vi "Stop Motion.vi"(4 "error in (no error)":errorcluster, 5 "Stop all axes (F)":bool, 6 "Axis (1)":i32=1 min=1 max=3, 7 "VISA resource name":refnum<visa-resource-name>) -> (0 "error out":errorcluster, 3 "VISA resource name out":refnum<visa-resource-name>)   [LabVIEW 2012, in "Newport ESP301.lvlib"]
doc: "This command stops a motion in progress using deceleration rate programmed with AG (set deceleration) command on the specified axes (or all axes if <B>Stop all axes (F)</B>=T)"
uses:
  Newport ESP301.lvlib
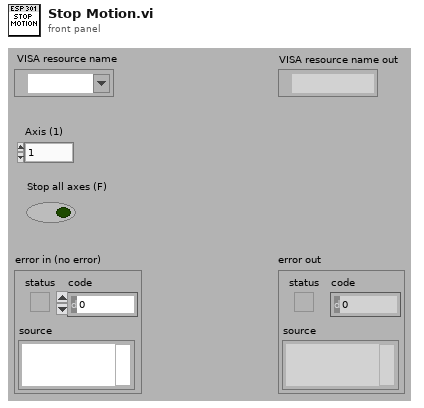
[diagram p1: front panel]
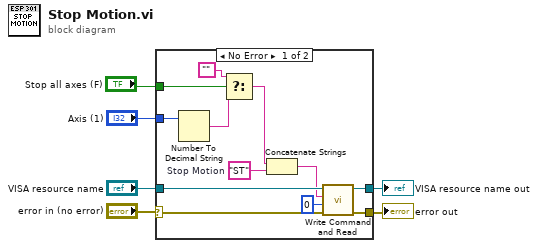
[diagram p0: block diagram]
diagram:
  n1 = case shown="No Error" "error in (no error)" {
    selector: "error in (no error)" -> [w15 w20]
    tunnel: [w17 w20] -> w6
    tunnel: "VISA resource name" -> [w18 w19]
    tunnel: [w16 w19] -> w5
    tunnel: "Axis (1)" -> [w12 _]
    tunnel: "Stop all axes (F)" -> [w10 _]
    frame No Error {
      w14 = "ST"  # Stop Motion
      n2 = Number To Decimal String(number=w12) -> (decimal integer string=w8:string)  [unwired: 1 in]
      n3 = Select(t="", s=w10, f=w8) -> (s? t:f=w9:string)
      n4 = Concatenate Strings(w9, w14) -> (w13:string)
      n5 = call "Write Command and Read.vi"("error in (no error)"=w15, "Bytes to read (100)"=u32 0, "Command"=w13, "VISA resource name"=w18) -> ("error out"=w17:errorcluster, "VISA resource name out"=w16:refnum<visa-resource-name>)  [unwired: 3 in, 1 out]
    }
    frame Error {
    }
  }
  "error out" <- w6
  "VISA resource name out" <- w5
